vi "JSON Unescape.vi"(8 "error in (no error)":errorcluster, 11 "Escaped String":string) -> (0 "error out":errorcluster, 2 "Characters Unescaped?":bool, 3 "String out":string)   [LabVIEW 2018, in "labview_json.lvlib"]
uses:
  labview_json.lvlib
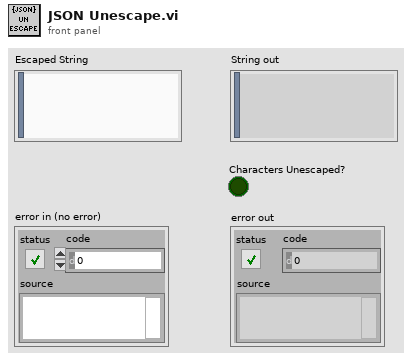
[diagram p1: front panel]
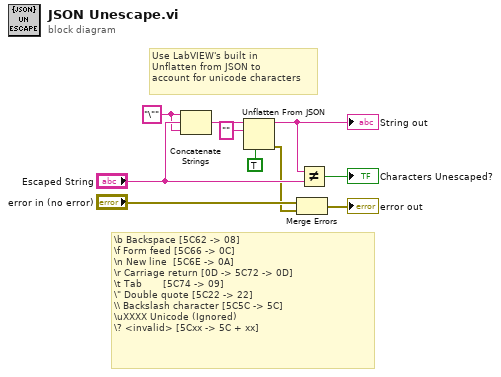
[diagram p0: block diagram]
diagram:
  w4 = "\"" ("string")
  # "Use LabVIEW's built in\nUnflatten from JSON to\naccount for unicode characters"
  # "\\b Backspace [5C62 -> 08]\n\\f Form feed [5C66 -> 0C]\n\\n New line  [5C6E -> 0A]\n\\r Carriage return [0D -> 5C72 -> 0D]\n\\t Tab       [5C74 -> 09]\n\\\" Double quote [5C22 -> 22]\n\\\\ Backslash character [5C5C -> 5C]\n\\uXXXX Unicode (Ignored)\n\\? <invalid> [5Cxx -> 5C + xx]"
  n1 = Concatenate Strings(w4, "Escaped String", w4) -> (w5:string)
  n2 = Unflatten From JSON(JSON string=w5, type and defaults="", default null elements? (F)=TRUE) -> (value=w9:string, error out=w2:errorcluster)  [unwired: 4 in]
  "String out" <- w9
  n3 = Merge Errors("error in (no error)", w2) -> (→"error out":errorcluster)
  n4 = Not Equal?(x=w9, y="Escaped String") -> (x != y?=→"Characters Unescaped?":bool)
